vi "InitializeDisplay (SubVI).vi"(8 "error in (no error)":errorcluster, 11 "Display Queue in":refnum<queue>) -> (0 "error out":errorcluster, 3 "Display Queue out":refnum<queue>)   [LabVIEW 2017]
doc: "Enqueues the appropiate commands to the Display Queue for initializing the front panel of the ATM application."
uses:
  Controls/DisplayControl.ctl
  Controls/DisplayCommand.ctl
  Controls/EnableDisableCommand.ctl
  Controls/UpdateMessageControl.ctl
  Controls/UpdateMessageCommand.ctl
  Controls/UpdateMenuCommand.ctl
  Controls/LedControl.ctl
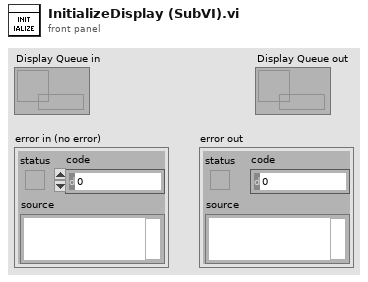
[diagram p1: front panel]
types:
  T1 = typedef "LedControl.ctl" = enum16{"Parcel0", "Parcel1", "Parcel2", "Parcel3", "Parcel4"}
  T2 = typedef "DisplayControl.ctl" = cluster{"Command":T3, "Data":variant}
  T3 = typedef "DisplayCommand.ctl" = enum16{"Initialize", "Open/Close Parcel", "Enable/Disable Controls", "FocusCursor", "UpdateMessage", "UpdateMenus", "FinishOperation", "Exit", "CleanUserInput"}
  T4 = typedef "UpdateMenuCommand.ctl" = enum16{"MainMenu", "NoMenu"}
  T5 = typedef "UpdateMessageControl.ctl" = cluster{"Command":T6, "Data":variant}
  T6 = typedef "UpdateMessageCommand.ctl" = enum16{"SystemCrash2", "SystemCrash1", "Welcome", "MainMenu", "PhoneNumberFailed", "PhoneNumberSuccess", "ParcelNumberSuccess", "ParcelNumbertFailed", "SessionTerminate", "SessionFinished", "Deposit", "DepositComplete", "Withdrawal", "WithdrawalComplete", "WithdrawalFailed"}
  T7 = typedef "EnableDisableCommand.ctl" = enum16{"InitialSetup", "StartOperation", "EnableUserInput", "DisableUserInput", "EnableMenus", "DisableMenus"}
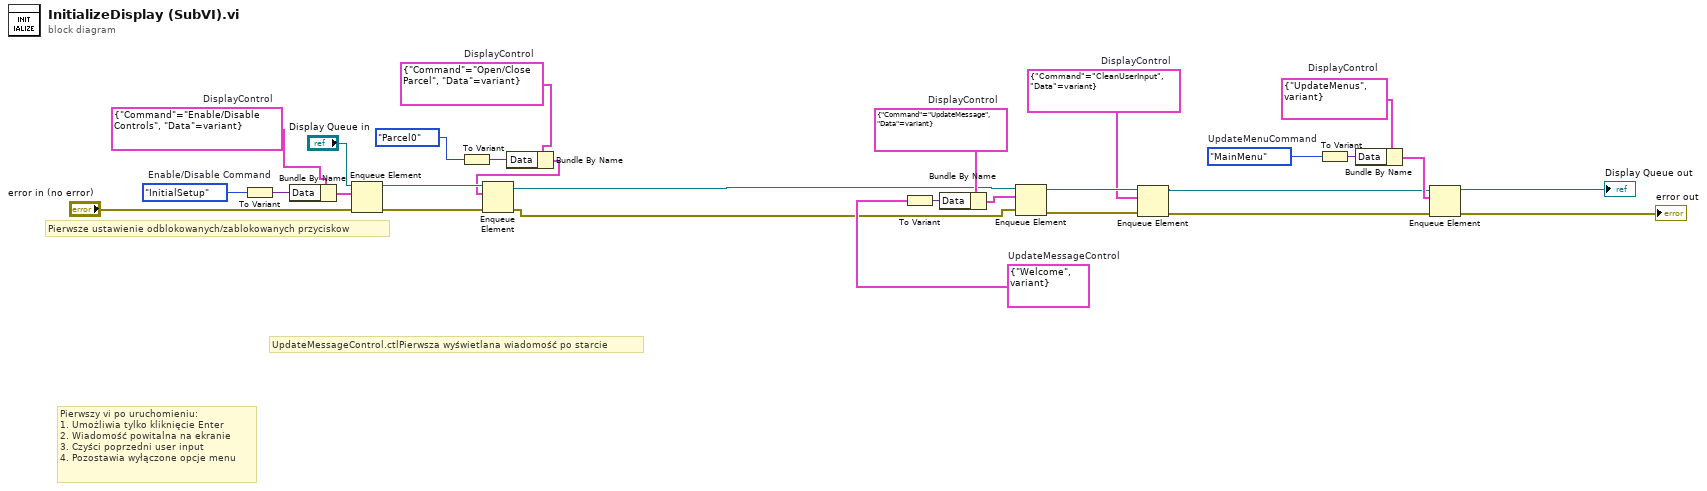
[diagram p0: block diagram]
diagram:
  w2 = T2 {"Command"=enum."Open/Close Parcel", "Data"=variant}  # DisplayControl
  w18 = T2 {"Command"=enum."UpdateMenus", "Data"=variant}  # DisplayControl
  w19 = UpdateMenuCommand."MainMenu"  # UpdateMenuCommand
  w20 = T2 {"Command"=enum."CleanUserInput", "Data"=variant}  # DisplayControl
  w23 = T5 {"Command"=enum."Welcome", "Data"=variant}  # UpdateMessageControl
  w24 = T2 {"Command"=enum."UpdateMessage", "Data"=variant}  # DisplayControl
  w29 = EnableDisableCommand."InitialSetup"  # Enable/Disable Command
  w11 = T2 {"Command"=enum."Enable/Disable Controls", "Data"=variant}  # DisplayControl
  # "Pierwszy vi po uruchomieniu:\n1. Umożliwia tylko kliknięcie Enter\n2. Wiadomość powitalna na ekranie\n3. Czyści poprzedni user input\n4. Pozostawia wyłączone opcje menu"
  # "Pierwsze ustawienie odblokowanych/zablokowanych przyciskow"
  # "UpdateMessageControl.ctlPierwsza wyświetlana wiadomość po starcie"
  n1 = To Variant(anything=w29) -> (Variant=w10:variant)
  n2 = Bundle By Name(cluster=w11, "Data"=w10) -> (w28:T2)
  n3 = Enqueue Element(queue="Display Queue in", element=w28, error in (no error)="error in (no error)") -> (queue out=w8:refnum<queue>, error out=w7:errorcluster)  [unwired: 1 in, 1 out]
  n4 = To Variant(anything=LedControl."Parcel0" ("MenuItem")) -> (Variant=w4:variant)
  n5 = Bundle By Name(cluster=w2, "Data"=w4) -> (w1:T2)
  n6 = Enqueue Element(queue=w8, element=w1, error in (no error)=w7) -> (queue out=w5:refnum<queue>, error out=w6:errorcluster)  [unwired: 1 in, 1 out]
  n7 = To Variant(anything=w23) -> (Variant=w26:variant)
  n8 = Bundle By Name(cluster=w24, "Data"=w26) -> (w25:T2)
  n9 = Enqueue Element(queue=w5, element=w25, error in (no error)=w6) -> (queue out=w21:refnum<queue>, error out=w22:errorcluster)  [unwired: 1 in, 1 out]
  n10 = Enqueue Element(queue=w21, element=w20, error in (no error)=w22) -> (queue out=w15:refnum<queue>, error out=w14:errorcluster)  [unwired: 1 in, 1 out]
  n11 = To Variant(anything=w19) -> (Variant=w16:variant)
  n12 = Bundle By Name(cluster=w18, "Data"=w16) -> (w17:T2)
  n13 = Enqueue Element(queue=w15, element=w17, error in (no error)=w14) -> (queue out=→"Display Queue out":refnum<queue>, error out=→"error out":errorcluster)  [unwired: 1 in, 1 out]
